vi "CalibratedMultipleMeasurements.vi"(7 "Show on call?":bool=TRUE, 8 "error in":errorcluster, 9 "Time between calibrations (ms)":u32=1000, 10 "Time / ms (30000)":u32=30000, 11 "VISA resource name":refnum<visa-resource-name>) -> (0 "error out":errorcluster, 1 "Times / LSB":dbl[](array[numeric]), 2 "Times / s":dbl[](array[numeric]), 3 "VISA resource name out":refnum<visa-resource-name>)   [LabVIEW 2018, in "GP22_TDC_Arduinoed.lvlib"]
doc: "Take measurements for the given amount of time, returning an array of doubles and handling calibration automatically."
uses:
  GP22_TDC_Arduinoed.lvlib
  <vilib>/Analysis/NI_AALPro.lvlib
panel:
  out "Histogram Graph":T1(graph)
  out "Calibration / LSB":dbl[](array[numeric])
  out "MMProgress":u8(slide) scale=0.0..100.0
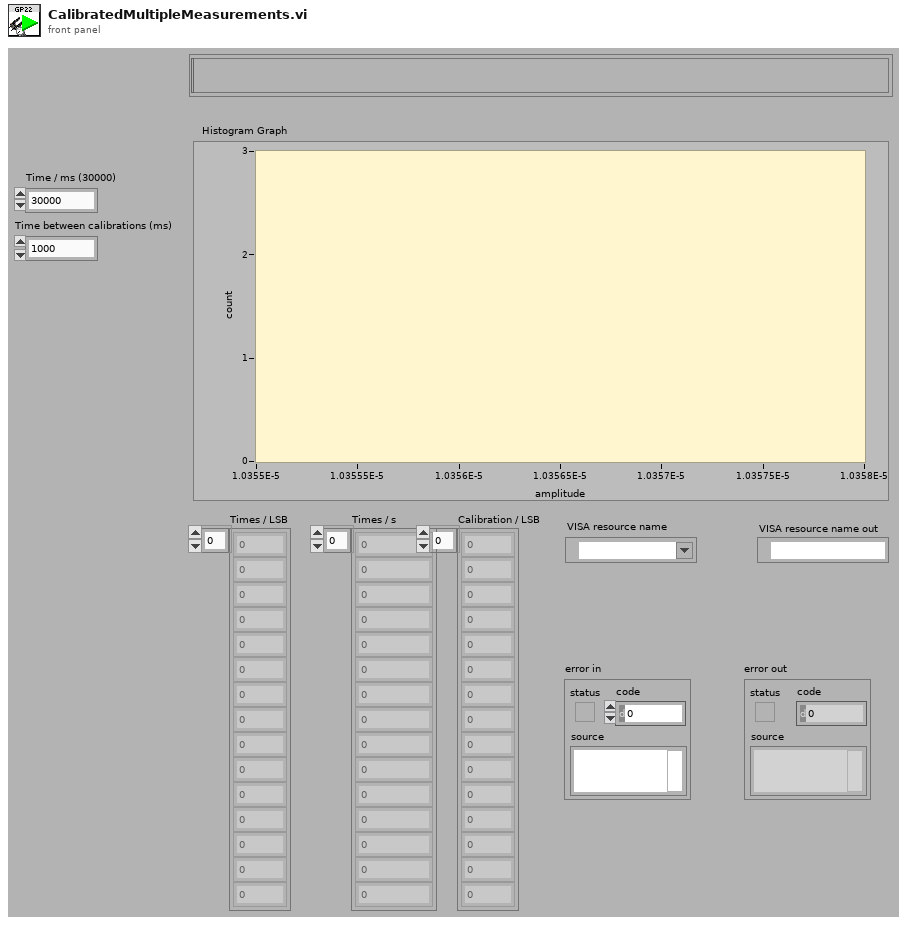
[diagram p1: front panel]
types:
  T1 = cluster{"X Values":dbl[], "Histogram: h(x)":i32[]}
  T2 = enum32{"Invalid", "Standard", "Closed", "Hidden", "Minimized", "Maximized"}
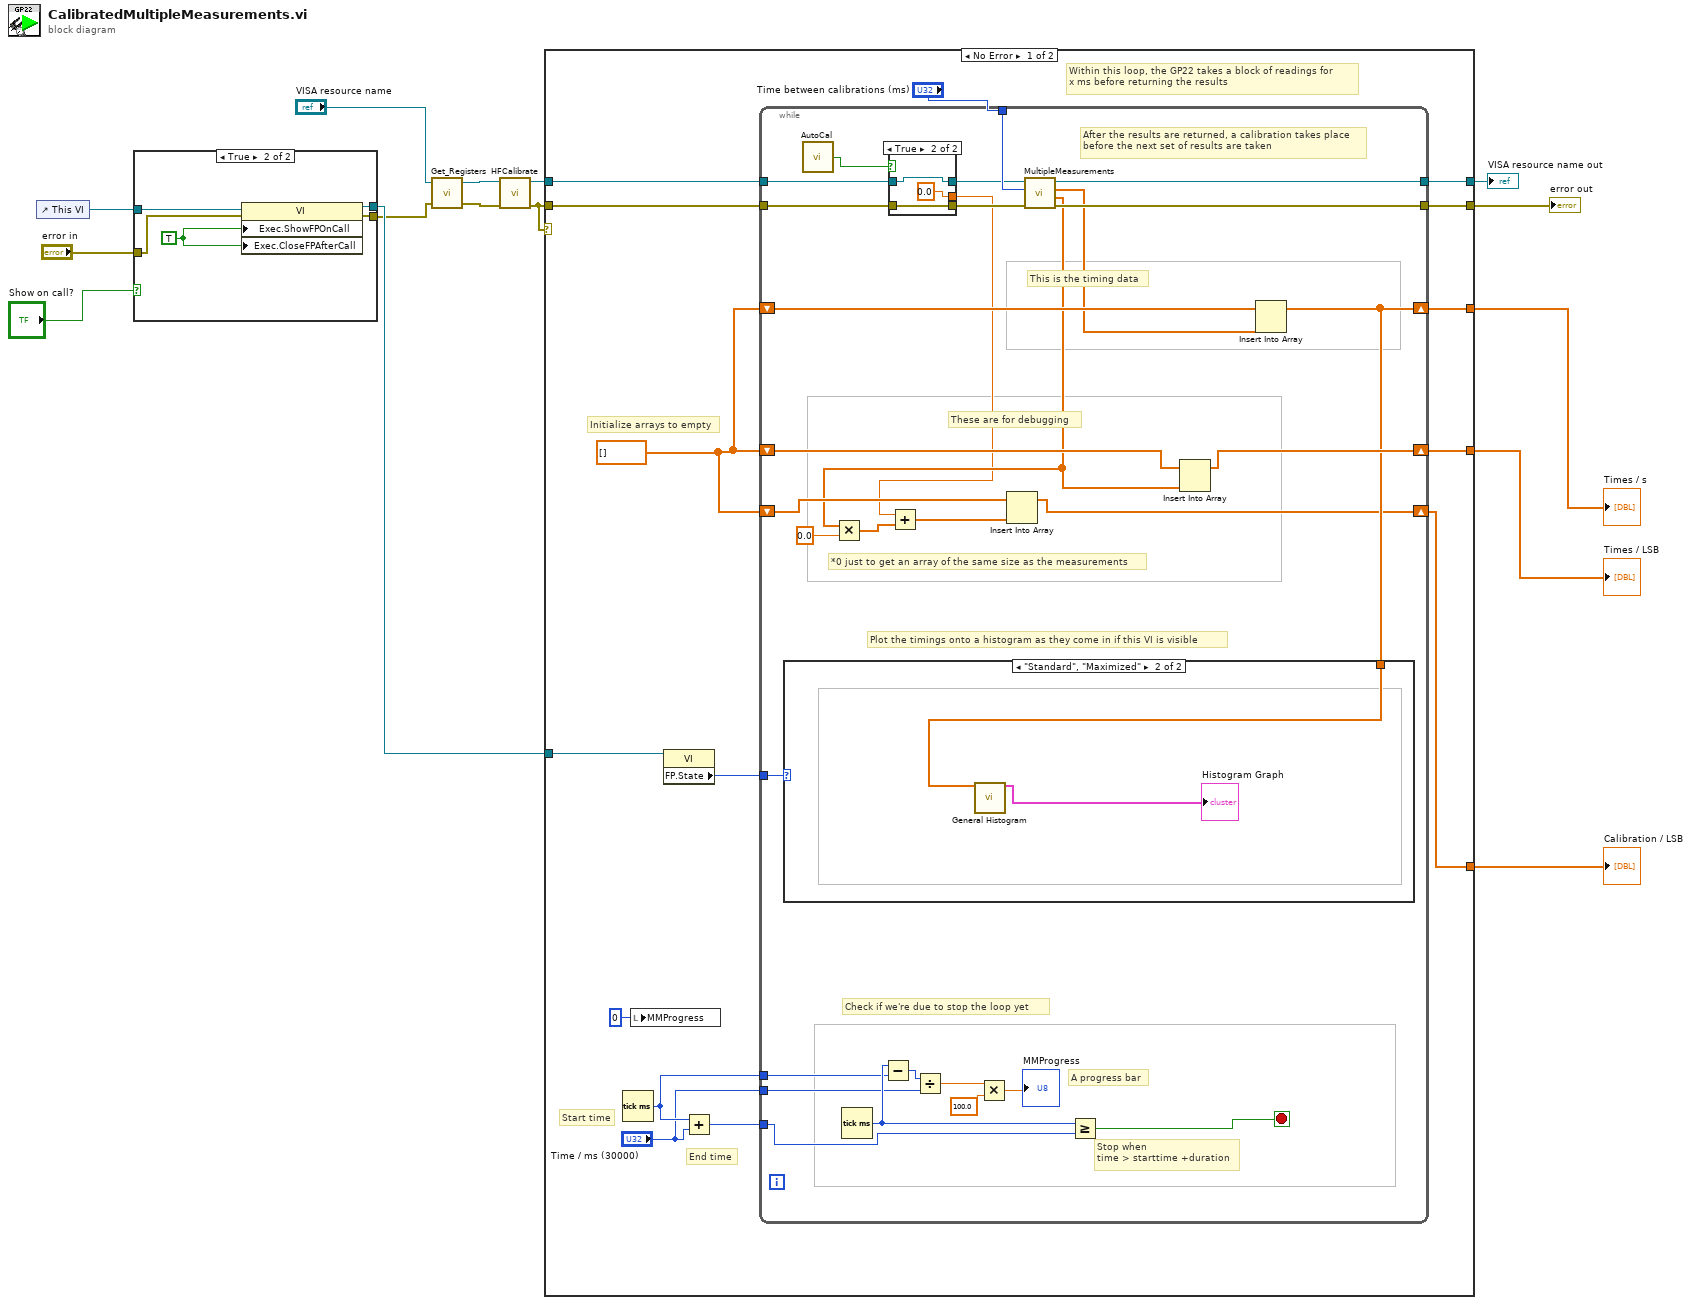
[diagram p0: block diagram]
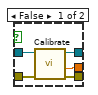
[diagram p3: hidden frame]
diagram:
  n1 = control-ref of="This VI"() -> (w9:refnum<vi>)
  n2 = case shown="True" "Show on call?" {
    tunnel: w9 -> [w16 w22]
    tunnel: [w16 w20] -> w8
    tunnel: "error in" -> [w17 w19]
    tunnel: [w17 w18] -> w1
    frame False {
    }
    frame True {
      w21 = TRUE ("Execution:Close After Call")
      n3 = property class="VI"(reference=w22, error in=w19, "Exec.ShowFPOnCall"=w21, "Exec.CloseFPAfterCall"=w21) -> (reference out=w20:refnum<vi>, error out=w18:errorcluster)
    }
  }
  n4 = call "Get_Registers.vi"("error in (no error)"=w1, "VISA in"="VISA resource name") -> ("error out"=w4:errorcluster, "VISA out"=w3:refnum<visa-resource-name>)  [unwired: 1 in, 1 out]
  n5 = call "HFCalibrate.vi"("error in (no error)"=w4, "VISA resource name"=w3) -> ("error out"=w5:errorcluster, "VISA resource name out"=w10:refnum<visa-resource-name>)  [unwired: 5 in, 2 out]
  n6 = case shown="No Error" w5 {
    tunnel: [w33 w79] -> w15
    tunnel: [w32 w78] -> w14
    tunnel: [w31 _] -> w13
    tunnel: [w30 _] -> w12
    tunnel: [w29 _] -> w11
    tunnel: w5 -> [w26 w78]
    tunnel: w10 -> [w25 w79]
    tunnel: w8 -> [w23 _]
    frame No Error {
      w28 = dbl[] []
      # "Initialize arrays to empty"
      # "Within this loop, the GP22 takes a block of readings for\nx ms before returning the results"
      # "End time"
      # "Start time"
      n7 = Tick Count (ms)() -> (millisecond timer value=w35:u32)
      n8 = local write "MMProgress"(u8 0 ("MMProgress")) -> ()
      n9 = property class="VI"(reference=w23) -> ("FP.State"=w27:T2)  [unwired: 1 in, 2 out]
      n10 = Add(x=w35, y="Time / ms (30000)") -> (x+y=w37:u32)
      n11 = while {
        tunnel: [w67] -> w33
        tunnel: "Time between calibrations (ms)" -> [w66]
        tunnel: w26 -> [w63]
        tunnel: [w65] -> w32
        tunnel: w37 -> [w50]
        shift-right: [w49] -> w31
        shift-left: w28 -> [w60]
        shift-right: [w57] -> w30
        shift-left: w28 -> [w58]
        shift-right: [w41] -> w29
        shift-left: w28 -> [w56]
        tunnel: w35 -> [w47]
        tunnel: "Time / ms (30000)" -> [w45]
        tunnel: w27 -> [w40]
        tunnel: w25 -> [w39]
        stop <- w64 stop-if-true
        # "Plot the timings onto a histogram as they come in if this VI is visible"
        # "Check if we're due to stop the loop yet"
        # "A progress bar"
        # "These are for debugging"
        # "This is the timing data"
        # "After the results are returned, a calibration takes place\nbefore the next set of results are taken"
        # "*0 just to get an array of the same size as the measurements"
        # "Stop when \ntime > starttime +duration"
        n12 = call "AutoCal.vi"() -> ("Autocal mode?"=w38:bool)  [unwired: 2 in]
        n13 = Tick Count (ms)() -> (millisecond timer value=w48:u32)
        n14 = Subtract(x=w48, y=w47) -> (x-y=w46:u32)
        n15 = case shown="True" w38 {
          tunnel: w63 -> [w74 w77]
          tunnel: [w73 w77] -> w62
          tunnel: [w72 w75] -> w61
          tunnel: [w71 0.0 ("y")] -> w52
          tunnel: w39 -> [w70 w75]
          frame False {
            n16 = call "Calibrate.vi"("error in (no error)"=w74, "VISA resource name"=w70) -> ("error out"=w73:errorcluster, "output raw"=w71:dbl, "VISA resource name out"=w72:refnum<visa-resource-name>)  [unwired: 5 in, 1 out]
          }
          frame True {
          }
        }
        n17 = Divide(x=w46, y=w45) -> (x/y=w44:dbl)
        n18 = Multiply(x=w44, y=100.0) -> (x*y=→"MMProgress":dbl)
        n19 = call "MultipleMeasurements.vi"("error in (no error)"=w62, "Time in ms (30000)"=w66, "VISA resource name"=w61) -> ("error out"=w65:errorcluster, "Raw output"=w55:dbl[], "output/s"=w59:dbl[], "VISA resource name out"=w67:refnum<visa-resource-name>)  [unwired: 5 in]
        n20 = Multiply(x=w55, y=0.0) -> (x*y=w53:dbl[])
        n21 = Add(x=w52, y=w53) -> (x+y=w51:dbl[])
        n22 = Insert Into Array(array=w56, new element=w51) -> (w41:dbl[])  [unwired: 1 in]
        n23 = Greater Or Equal?(x=w48, y=w50) -> (x >= y?=w64:bool)
        n24 = Insert Into Array(array=w58, new element=w55) -> (w57:dbl[])  [unwired: 1 in]
        n25 = Insert Into Array(array=w60, new element=w59) -> (w49:dbl[])  [unwired: 1 in]
        n26 = case shown="\"Standard\", \"Maximized\"" w40 {
          tunnel: w49 -> [_ w69]
          frame "Invalid", Default {
            # "Do nothing here if this VI isn't visible"
          }
          frame "Standard", "Maximized" {
            n27 = call <vilib>:"General Histogram.vi"("X"=w69) -> ("Histogram Graph"=→"Histogram Graph":T1)  [unwired: 10 in, 4 out]
          }
        }
      }
    }
    frame Error {
    }
  }
  "VISA resource name out" <- w15
  "error out" <- w14
  "Times / s" <- w13
  "Times / LSB" <- w12
  "Calibration / LSB" <- w11
